vi "get_data_from_control_string.vi"(8 "error in":errorcluster, 10 "control label":string, 11 "controls array":refnum<vi>[](array[refnum])) -> (0 "error out":errorcluster, 3 "string out":string)   [LabVIEW 2019]
panel:
  out "all labels":string[](array[string])
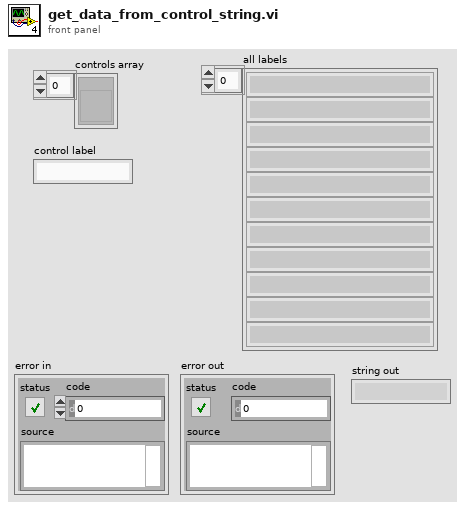
[diagram p1: front panel]
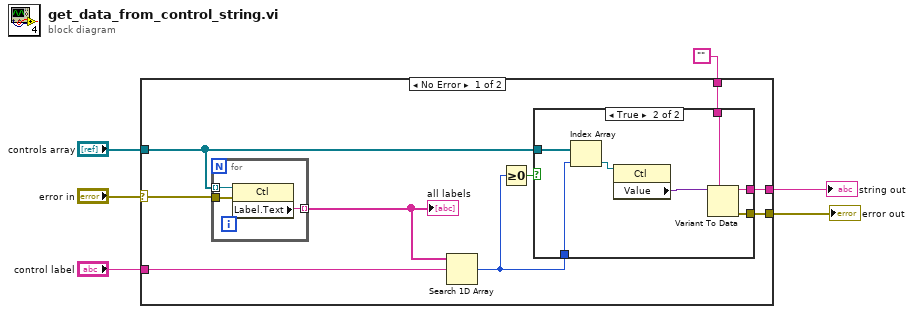
[diagram p0: block diagram]
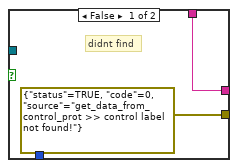
[diagram p2: hidden frame]
diagram:
  n1 = case shown="No Error" "error in" {
    selector: "error in" -> [w10 w29]
    tunnel: "control label" -> [w15 _]
    tunnel: "controls array" -> [w13 _]
    tunnel: [w12 w28] -> w1
    tunnel: [w11 w29] -> w5
    tunnel: "" -> [w7 w28]
    frame No Error {
      n2 = for {
        tunnel: w13 -> [w27] mode=indexing
        tunnel: [w26] -> w14 mode=indexing
        tunnel: w10 -> [w25]
        n3 = property class="Ctl"(reference=w27, error in=w25) -> ("Label.Text"=w26:string)  [unwired: 2 out]
      }
      "all labels" <- w14
      n4 = Search 1D Array(1D array=w14, element=w15) -> (index of element=w8:i32)  [unwired: 1 in]
      n5 = Greater Or Equal To 0?(x=w8) -> (x >= 0?=w9:bool)
      n6 = case shown="True" w9 {
        tunnel: w13 -> [_ w24]
        tunnel: w8 -> [_ w23]
        tunnel: [w16 w22] -> w12
        tunnel: [errorcluster {"status"=TRUE, "code"=0, "source"="get_data_from_control_prot >> control label not found!"} ("error out") w19] -> w11
        tunnel: w7 -> [w16 w18]
        frame False {
          # "didnt find"
        }
        frame True {
          n7 = Index Array(array=w24, index=w23) -> (element=w21:refnum<vi>)
          n8 = property class="Ctl"(reference=w21) -> ("Value"=w20:variant)  [unwired: 1 in, 2 out]
          n9 = Variant To Data(type=w18, Variant=w20) -> (data=w22:string, error out=w19:errorcluster)  [unwired: 1 in]
        }
      }
    }
    frame Error {
    }
  }
  "error out" <- w5
  "string out" <- w1
